vi "Restore Commas to Data.vi"(3 "Data In":string[][](array[string])) -> (6 "Data Out":string[][](array[string]))   [LabVIEW 2013]
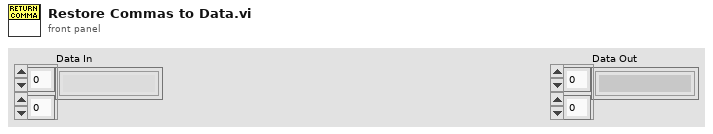
[diagram p1: front panel]
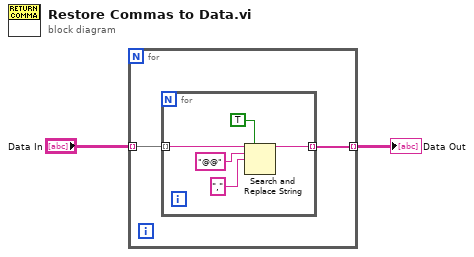
[diagram p0: block diagram]
diagram:
  n1 = for {
    tunnel: "Data In" -> [w4] mode=indexing
    tunnel: [w3] -> w1 mode=indexing
    n2 = for {
      tunnel: w4 -> [w9] mode=indexing
      tunnel: [w5] -> w3 mode=indexing
      n3 = Search and Replace String(replace all?=TRUE ("replace all? (F)"), input string=w9, search string="@@", replace string="," ("replace string (\"\")")) -> (result string=w5:string)  [unwired: 4 in, 3 out]
    }
  }
  "Data Out" <- w1
